vi "JYGetMonos.vi"(1 "error in (no error)":errorcluster) -> (2 "UniqueIDs":string[](array[string]), 3 "Names":string[](array[string]), 5 "error out":errorcluster)   [LabVIEW 2009]
doc: "JYGetMonos.vi\nInput - Input Error Cluster\n----------------------------------\n\nOutputs -\nUniquedIDs - string array\nDisplayNames - string array\nOutput Error Cluster\n\nUses the JYConfiguration Browser return a list\nof registered monos.\n\nThe UniqueID will be required to initialize\nthe mono"
panel:
  in  "Monos":i32(listbox)
  in  "Config Browser":refnum<k7>
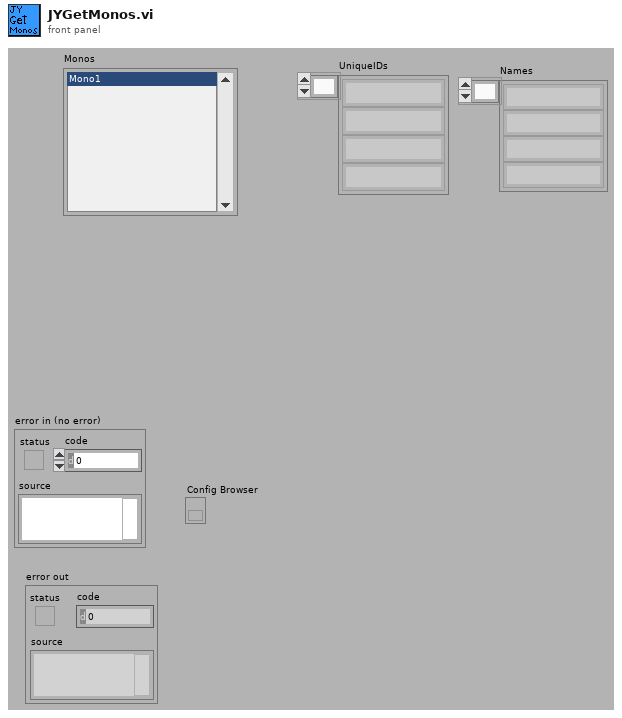
[diagram p1: front panel]
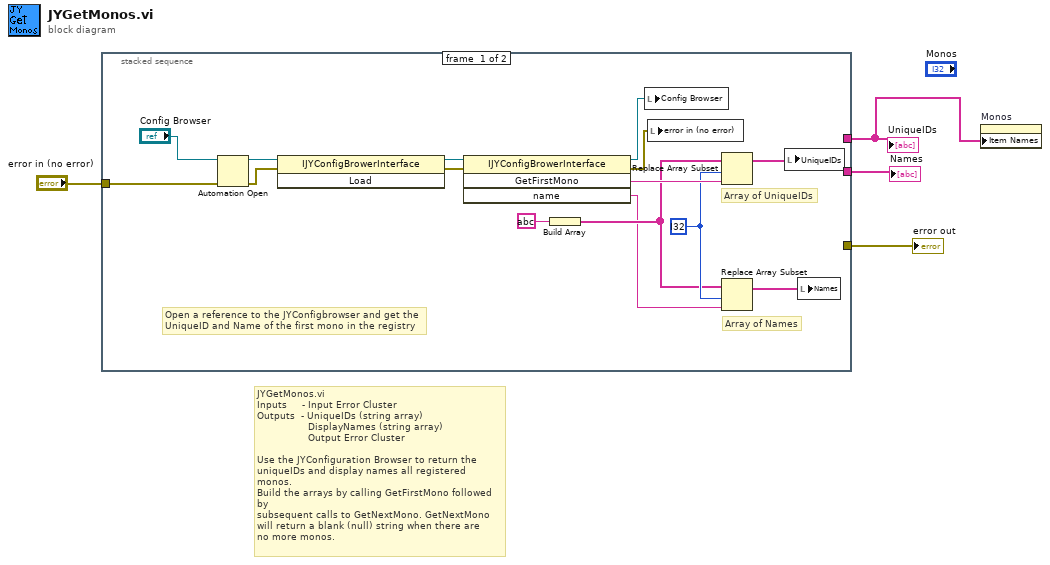
[diagram p0: block diagram]
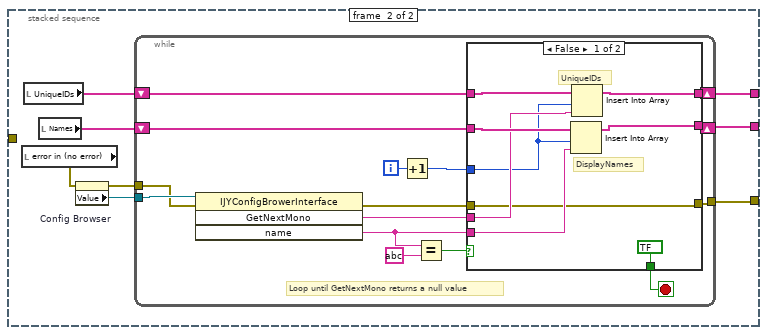
[diagram p2: hidden frame]
diagram:
  # "JYGetMonos.vi\nInputs     - Input Error Cluster\nOutputs  - UniqueIDs (string array)\n                 DisplayNames (string array)\n                 Output Error Cluster\n\nUse the JYConfiguration Browser to return the\nuniqueIDs and display names all registered monos.\nBuild the arrays by calling GetFirstMono followed by\nsubsequent calls to GetNextMono. GetNextMono\nwill return a blank (null) string when there are\nno more monos."
  n1 = stacked-sequence {
    tunnel: [_ w22] -> w3
    tunnel: [_ w21] -> w4
    tunnel: [_ w20] -> w1
    tunnel: "error in (no error)" -> [w5 _]
    frame #0 {
      w10 = i32 ?
      # "Array of Names"
      # "Array of UniqueIDs"
      # "Open a reference to the JYConfigbrowser and get the\nUniqueID and Name of the first mono in the registry"
      n2 = Automation Open(error in (no error)=w5, Automation Refnum="Config Browser") -> (Automation Refnum=w19:refnum<k7>, error out=w17:errorcluster)  [unwired: 2 out]
      n3 = invoke class="IJYConfigBrowerInterface" method="Load"(reference=w19, error in=w17) -> (reference out=w18:refnum<k7>, error out=w16:errorcluster)  [unwired: 1 in, 1 out]
      n4 = invoke class="IJYConfigBrowerInterface" method="GetFirstMono"(reference=w18, error in=w16) -> (reference out=w14:refnum<k7>, error out=w12:errorcluster, "GetFirstMono"=w11:string, "name"=w8:string)  [unwired: 2 in]
      n5 = Build Array(string ?) -> (w9:string[])
      n6 = local write "Config Browser"(w14) -> ()
      n7 = local write "error in (no error)"(w12) -> ()
      n8 = Replace Array Subset(array=w9, new element=w11, index=w10) -> (w7:string[])
      n9 = Replace Array Subset(array=w9, new element=w8, index=w10) -> (w6:string[])
      n10 = local write "UniqueIDs"(w7) -> ()
      n11 = local write "Names"(w6) -> ()
    }
    frame #1 {
      n12 = local read "error in (no error)"() -> (w26:errorcluster)
      n13 = local read "UniqueIDs"() -> (w24:string[])
      n14 = local read "Names"() -> (w23:string[])
      n15 = property on="Config Browser" class="Ref (strict)"(error in=w26) -> (error out=w25:errorcluster, "Value"=w27:refnum<k7>)  [unwired: 1 in, 1 out]
      n16 = while {
        tunnel: w27 -> [w42]
        tunnel: w25 -> [w41]
        shift-right: [w28] -> w22
        shift-left: w24 -> [w29]
        shift-right: [w35] -> w21
        shift-left: w23 -> [w36]
        tunnel: [w30] -> w20
        i -> [w40]
        stop <- w37 stop-if-true
        # "Loop until GetNextMono returns a null value"
        n17 = invoke class="IJYConfigBrowerInterface" method="GetNextMono"(reference=w42, error in=w41) -> (error out=w31:errorcluster, "GetNextMono"=w34:string, "name"=w33:string)  [unwired: 2 in, 1 out]
        n18 = Increment(x=w40) -> (x+1=w32:i32)
        n19 = Equal?(x=w33, y=string ?) -> (x = y?=w38:bool)
        n20 = case shown="False" w38 {
          selector: w38 -> [_ w55]
          tunnel: [bool ? w55] -> w37
          tunnel: w29 -> [w44 w53]
          tunnel: w36 -> [w50 w52]
          tunnel: [w46 w52] -> w35
          tunnel: w34 -> [w49 _]
          tunnel: w33 -> [w48 _]
          tunnel: w32 -> [w47 _]
          tunnel: w31 -> [w45 w54]
          tunnel: [w45 w54] -> w30
          tunnel: [w43 w53] -> w28
          frame #0 {
            # "DisplayNames"
            # "UniqueIDs"
            n21 = Insert Into Array(array=w50, index=w47, new element=w48) -> (w46:string[])
            n22 = Insert Into Array(array=w44, index=w47, new element=w49) -> (w43:string[])
          }
          frame #1 {
            # "Null value returned -\nno more monos - quit"
          }
        }
      }
    }
  }
  "UniqueIDs" <- w3
  "Names" <- w4
  "error out" <- w1
  n23 = property on="Monos" class="LstBox (strict)"("Item Names"=w3) -> ()  [unwired: 2 in, 2 out]
